vi "Get Routing Channel State Configurations.vi"(8 "error in":errorcluster, 11 "routing channel in":T4 format="%.0x") -> (0 "error out":errorcluster, 2 "state configurations":T1, 3 "routing channel out":T4=18446744073709551615 format="%.0x")   [LabVIEW 2020, in "Routing and Faulting Scripting.lvlib"]
doc: "Returns the states for the routing channel."
uses:
  Routing and Faulting Scripting.lvlib
  <vilib>/NI VeriStand/Custom Device API/Custom Device Item Ref.ctl
  Shared/Channel States.ctl
  Shared/Routing State.ctl
  Shared/Connection.ctl
  NationalInstruments.VeriStand.SystemDefinitionAPI
  Constants/Scripting Constants.vi
  Shared/Routing and Faulting Shared.lvlib
  <vilib>/NI VeriStand/Custom Device API/Custom Device API.lvlib
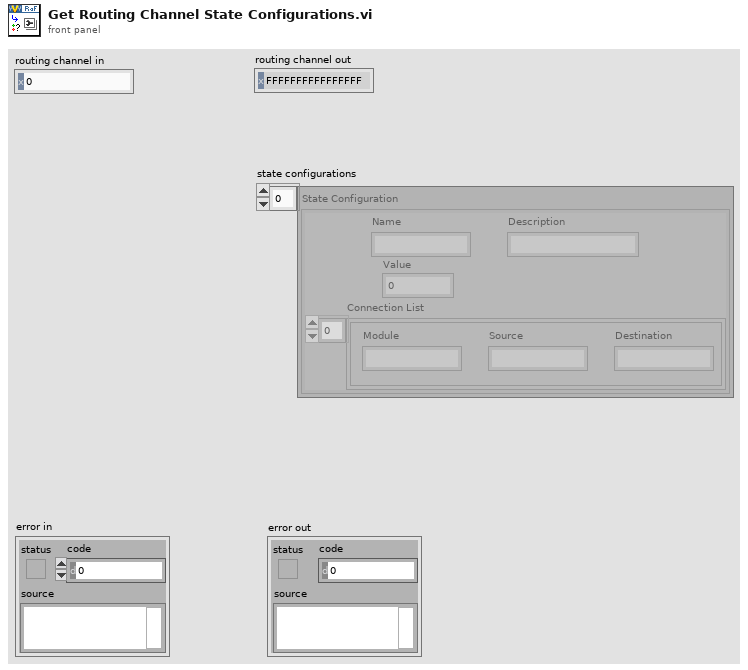
[diagram p1: front panel]
types:
  T1 = typedef "Routing and Faulting Shared.lvlib/Channel States.ctl" = T2[]
  T2 = typedef "Routing and Faulting Shared.lvlib/Routing State.ctl" = cluster{"Name":string, "Description":string, "Value":i32, "Connection List":T3[]}
  T3 = typedef "Routing and Faulting Shared.lvlib/Connection.ctl" = cluster{"Module":string, "Source":string, "Destination":string}
  T4 = typedef "Custom Device API.lvlib/Custom Device Item Ref.ctl" = u64
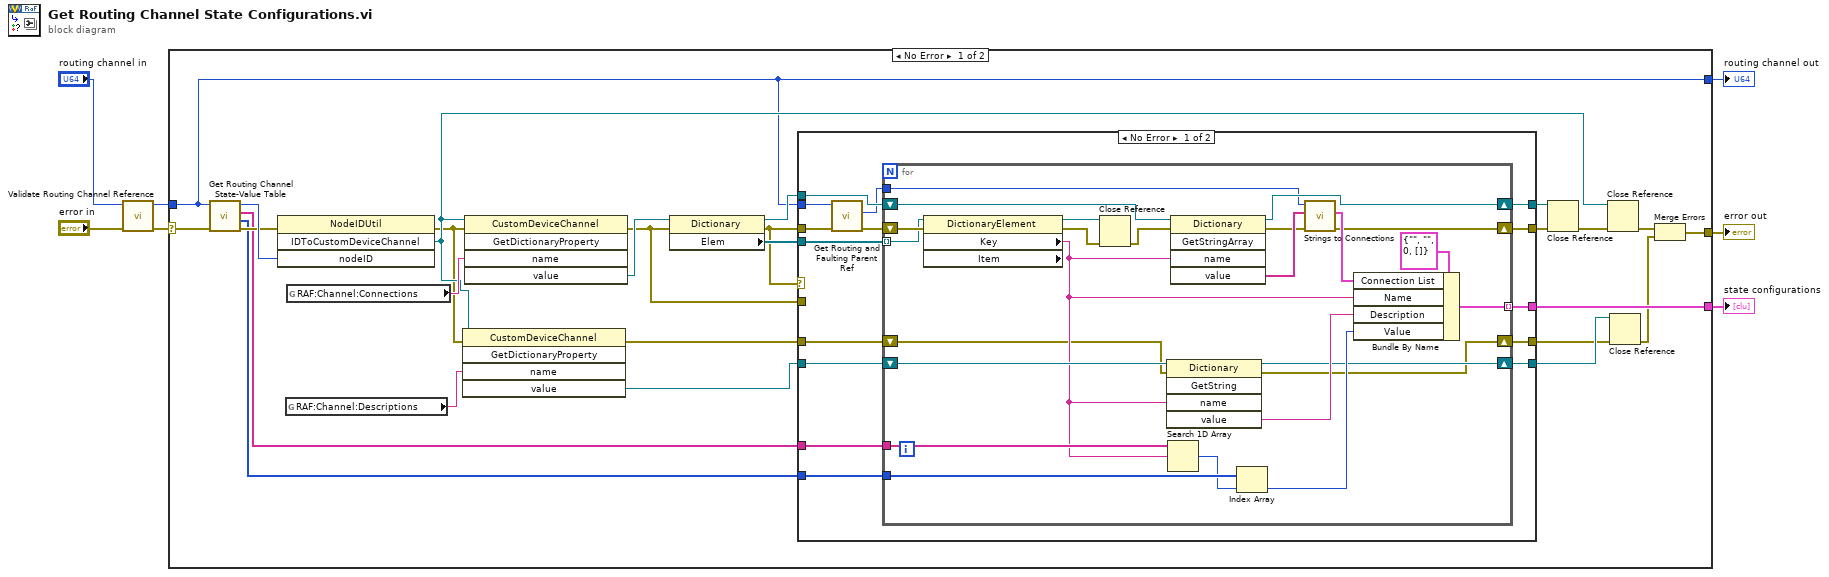
[diagram p0: block diagram]
diagram:
  n1 = call "Validate Routing Channel Reference.vi"("error in"="error in", "routing channel in"="routing channel in") -> ("error out"=w3:errorcluster, "routing channel out"=w1:T4)  [unwired: 8 in]
  n2 = case shown="No Error" w3 {
    selector: w3 -> [w29 w78]
    tunnel: [w12 w78] -> w6
    tunnel: w1 -> [w8 w77]
    tunnel: [w8 w77] -> w5
    tunnel: [w31 _] -> w4
    frame No Error {
      n3 = call "Get Routing Channel State-Value Table.vi"("error in"=w29, "routing channel in"=w8) -> ("error out"=w28:errorcluster, "state values"=w26:i32[], "state names"=w27:string[], "routing channel out"=w30:T4)  [unwired: 6 in]
      n4 = invoke class="NodeIDUtil" method="IDToCustomDeviceChannel"(error in=w28, "nodeID"=w30) -> (error out=w18:errorcluster, "IDToCustomDeviceChannel"=w21:refnum<k24>)  [unwired: 2 in, 2 out]
      n5 = global read "Scripting Constants.vi" "RAF:Channel:Descriptions"() -> (w22:string)
      n6 = global read "Scripting Constants.vi" "RAF:Channel:Connections"() -> (w25:string)
      n7 = invoke class="CustomDeviceChannel" method="GetDictionaryProperty"(reference=w21, error in=w18, "name"=w22) -> (error out=w17:errorcluster, "value"=w20:refnum<k24>)  [unwired: 2 in, 3 out]
      n8 = invoke class="CustomDeviceChannel" method="GetDictionaryProperty"(reference=w21, error in=w18, "name"=w25) -> (error out=w9:errorcluster, "value"=w32:refnum<k24>)  [unwired: 2 in, 3 out]
      n9 = property class="Dictionary"(reference=w32, error in=w9) -> (reference out=w11:refnum<k24>, error out=w10:errorcluster, "Elem"=w23:refnum<k24>[])
      n10 = case shown="No Error" w10 {
        tunnel: [w48 w75] -> w33
        tunnel: w11 -> [w47 w76]
        tunnel: [w46 _] -> w31
        tunnel: w27 -> [w45 _]
        tunnel: w26 -> [w44 _]
        tunnel: w10 -> [w43 _]
        tunnel: [w42 w76] -> w24
        tunnel: w23 -> [w41 _]
        tunnel: w20 -> [w40 w73]
        tunnel: [w39 w73] -> w19
        tunnel: w17 -> [w38 w74]
        tunnel: [w37 w74] -> w16
        tunnel: w9 -> [_ w75]
        tunnel: w8 -> [w35 _]
        frame No Error {
          n11 = call "Get Routing and Faulting Parent Ref.vi"("error in"=w43, "routing and faulting child in"=w35) -> ("error out"=w36:errorcluster, "routing and faulting"=w34:T4)  [unwired: 7 in, 1 out]
          n12 = for {
            shift-right: [w50] -> w48
            shift-left: w36 -> [w69]
            shift-right: [w59] -> w42
            shift-left: w47 -> [w64]
            tunnel: w41 -> [w68] mode=indexing
            tunnel: [w72] -> w46 mode=indexing
            tunnel: w45 -> [w71]
            tunnel: w44 -> [w70]
            shift-right: [w56] -> w39
            shift-left: w40 -> [w58]
            shift-right: [w54] -> w37
            shift-left: w38 -> [w55]
            tunnel: w34 -> [w49]
            n13 = property class="DictionaryElement" props=["Key", "Item"](reference=w68, error in=w69) -> (reference out=w67:refnum<k24>, error out=w66:errorcluster, "Key"=w57:string)  [unwired: 1 out]
            n14 = Close Reference(reference=w67, error in (no error)=w66) -> (error out=w65:errorcluster)
            n15 = invoke class="Dictionary" method="GetString"(reference=w58, error in=w55, "name"=w57) -> (reference out=w56:refnum<k24>, error out=w54:errorcluster, "value"=w60:string)  [unwired: 2 in, 2 out]
            n16 = Search 1D Array(1D array=w71, element=w57) -> (index of element=w62:i32)  [unwired: 1 in]
            n17 = invoke class="Dictionary" method="GetStringArray"(reference=w64, error in=w65, "name"=w57) -> (reference out=w59:refnum<k24>, error out=w51:errorcluster, "value"=w53:string[])  [unwired: 2 in, 2 out]
            n18 = Index Array(array=w70, index=w62) -> (element=w61:i32)
            n19 = call "Strings to Connections.vi"("error in"=w51, "connection strings"=w53, "routing and faulting in"=w49) -> ("error out"=w50:errorcluster, "connection list"=w52:T3[])  [unwired: 6 in, 1 out]
            n20 = Bundle By Name(cluster=T2 {"Name"="", "Description"="", "Value"=0, "Connection List"=[]} ("Routing State"), "Connection List"=w52, "Name"=w57, "Description"=w60, "Value"=w61) -> (w72:T2)
          }
        }
        frame Error {
          # "Dictionary exists, but their are no elements at this point\nNo Connections have been added to the Dictionary."
        }
      }
      n21 = Close Reference(reference=w24, error in (no error)=w33) -> (error out=w15:errorcluster)
      n22 = Close Reference(reference=w21, error in (no error)=w15) -> (error out=w14:errorcluster)
      n23 = Close Reference(reference=w19, error in (no error)=w16) -> (error out=w13:errorcluster)
      n24 = Merge Errors(w14, w13) -> (w12:errorcluster)
    }
    frame Error {
    }
  }
  "routing channel out" <- w5
  "error out" <- w6
  "state configurations" <- w4
